vi "Pfeiffer Vacuum OnTool Miscellaneous.vi"(8 "error in (no error)":errorcluster, 9 "PV OnTool Miscellaneous - Cluster":T1={"Parameter"=0, "Parameter\nread only<->describe"=FALSE, "Unit adress"=1, "Configuration output K1"=0, "Remote operations mode"=0, "Characteristic analog input "=0} {"Characteristic analog input" items=[" proportional rotation speed", " proportional rotation speed  <=15%", " proportional rotation speed >= 80%"]; "Remote operations mode" items=[" operations via remote", " operations via PV-Protocol"]; "Configuration output K1" items=[" User controlled", " Drive synchron", " Drive invers synchron"]; "Unit adress" min=1 max=255 step=1; "Parameter" items=[" Configuration output K1", " Remote operations mode", " Characteristic analog input", " Actual error code (read only)", " Software version electronic drive unit  (read only)", " Interlock ok  (read only)", " Unit type electronic drive unit", " Software version controller (read only)", " Hardware version (read only)", " Unit address", " Error acknowledgement"]}, 10 "Adress of unit":u16=1 min=1 max=999 step=1, 11 "COM Port Name in":refnum<visa-resource-name>="COM1") -> (0 "error out":errorcluster, 1 "response (data)":string)   [LabVIEW 2021]
doc: "This VI is an example of how to use the Pfeiffer Vacuum subVIs programmatically. This VI first initializes the instrument, takes measurements, then closes the instrument."
uses:
  <instrlib>/Pfeiffer Vacuum/Public/OnTool/PV OnTool Miscelaneous - Cluster.ctl
  <instrlib>/Pfeiffer Vacuum/Pfeiffer Vacuum.lvlib
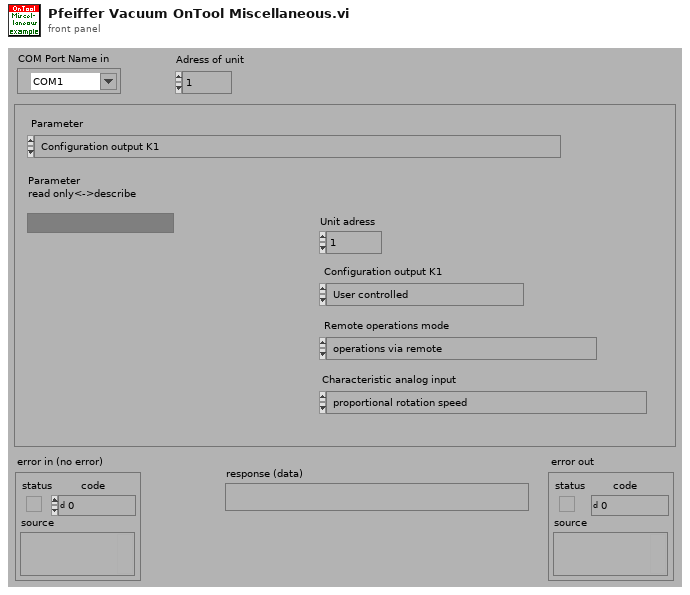
[diagram p1: front panel]
types:
  T1 = typedef "Pfeiffer Vacuum.lvlib/PV OnTool Miscelaneous - Cluster.ctl" = cluster{"Parameter":u16, "Parameter\nread only<->describe":bool, "Unit adress":i16, "Configuration output K1":u16, "Remote operations mode":u16, "Characteristic analog input ":u16}
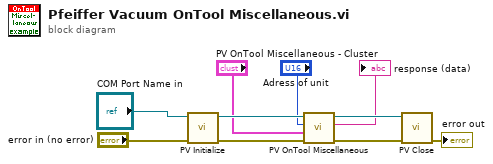
[diagram p0: block diagram]
diagram:
  n1 = call <instrlib>:"PV Initialize.vi"("error in (no error)"="error in (no error)", "VISA session in"="COM Port Name in") -> ("error out"=w5:errorcluster, "VISA session out"=w10:refnum<visa-resource-name>)  [unwired: 8 in]
  n2 = call <instrlib>:"PV OnTool Miscellaneous.vi"("error in (no error)"=w5, "PV OnTool Miscellaneous - Cluster"="PV OnTool Miscellaneous - Cluster", "Adress of unit"="Adress of unit", "VISA session"=w10) -> ("error out"=w4:errorcluster, "response (data)"=→"response (data)":string, "dup VISA session"=w9:refnum<visa-resource-name>)  [unwired: 5 in]
  n3 = call <instrlib>:"PV Close.vi"("VISA session"=w9, "error in (no error)"=w4) -> ("error out"=→"error out":errorcluster)  [unwired: 13 in]
